vi "Swervepostprossesing(mine) (SubVI).vi"(7 "Total ticks in rotation":dbl, 9 "Speed in":dbl, 10 "Angle in":dbl, 11 "refnum name":string="Steering FR") -> (0 "Boolean":bool=TRUE, 1 "Speed out":dbl, 2 "position":dbl, 3 "refnum name":string="Steering FR")   [LabVIEW 2020]
uses:
  <vilib>/Rock Robotics/WPI/ThirdParty/Phoenix-LabVIEW/Motor Controller/Get/CTRE_Phoenix_MotorController_GetSelectedSensorData.vi
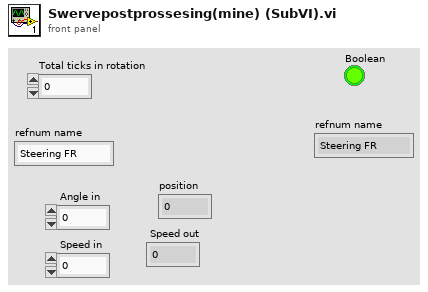
[diagram p1: front panel]
types:
  T1 = typedef "WPI_MotorControlDeviceRef.ctl" = cluster{"DeviceStatus":errorcluster, "Type":T2, "PWM":cluster{"PWM Channel":T3, "DeadBand":T4}, "CAN":cluster{"Device Number":u8, "SetOutput VI Ref":variant, "GetOutput VI Ref":variant, "Enable VI Ref":variant, "Disable VI Ref":variant, "Data":variant}, "Invert":bool, "DIO PWM":cluster{"PWM \"Enable\" Channel":T3, "DIOChannel":T5, "PWM Rate":dbl}}
  T2 = typedef "WPI_MotorControlType.ctl" = enum16{"PWM", "CAN", "DIO PWM"}
  T3 = typedef "FPGA_DIOPWMChannel.ctl" = enum8{"PWM 0", "PWM 1", "PWM 2", "PWM 3", "PWM 4", "PWM 5", "PWM 6", "PWM 7", "PWM 8", "PWM 9", "PWM MXP 0", "PWM MXP 1", "PWM MXP 2", "PWM MXP 3", "PWM MXP 4", "PWM MXP 5", "PWM MXP 6", "PWM MXP 7", "PWM MXP 8", "PWM MXP 9", "Invalid"}
  T4 = typedef "WPI_PWMDeadband.ctl" = cluster{"Name":string, "maxPositivePwm":i32, "minPositivePwm":i32, "centerPwm":i32, "maxNegativePwm":i32, "minNegativePwm":i32, "angularRange":u16}
  T5 = typedef "FPGA_DIOChannel.ctl" = enum8{"DIO 0", "DIO 1", "DIO 2", "DIO 3", "DIO 4", "DIO 5", "DIO 6", "DIO 7", "DIO 8", "DIO 9", "DIO MXP 0", "DIO MXP 1", "DIO MXP 2", "DIO MXP 3", "DIO MXP 4", "DIO MXP 5", "DIO MXP 6", "DIO MXP 7", "DIO MXP 8", "DIO MXP 9", "DIO MXP 10", "DIO MXP 11", "DIO MXP 12", "DIO MXP 13", "DIO MXP 14", "DIO MXP 15", "SPI Port CS1", "SPI Port CS2", "SPI Port CS3", "SPI Port MISO", "SPI Port MOSI", "Invalid"}
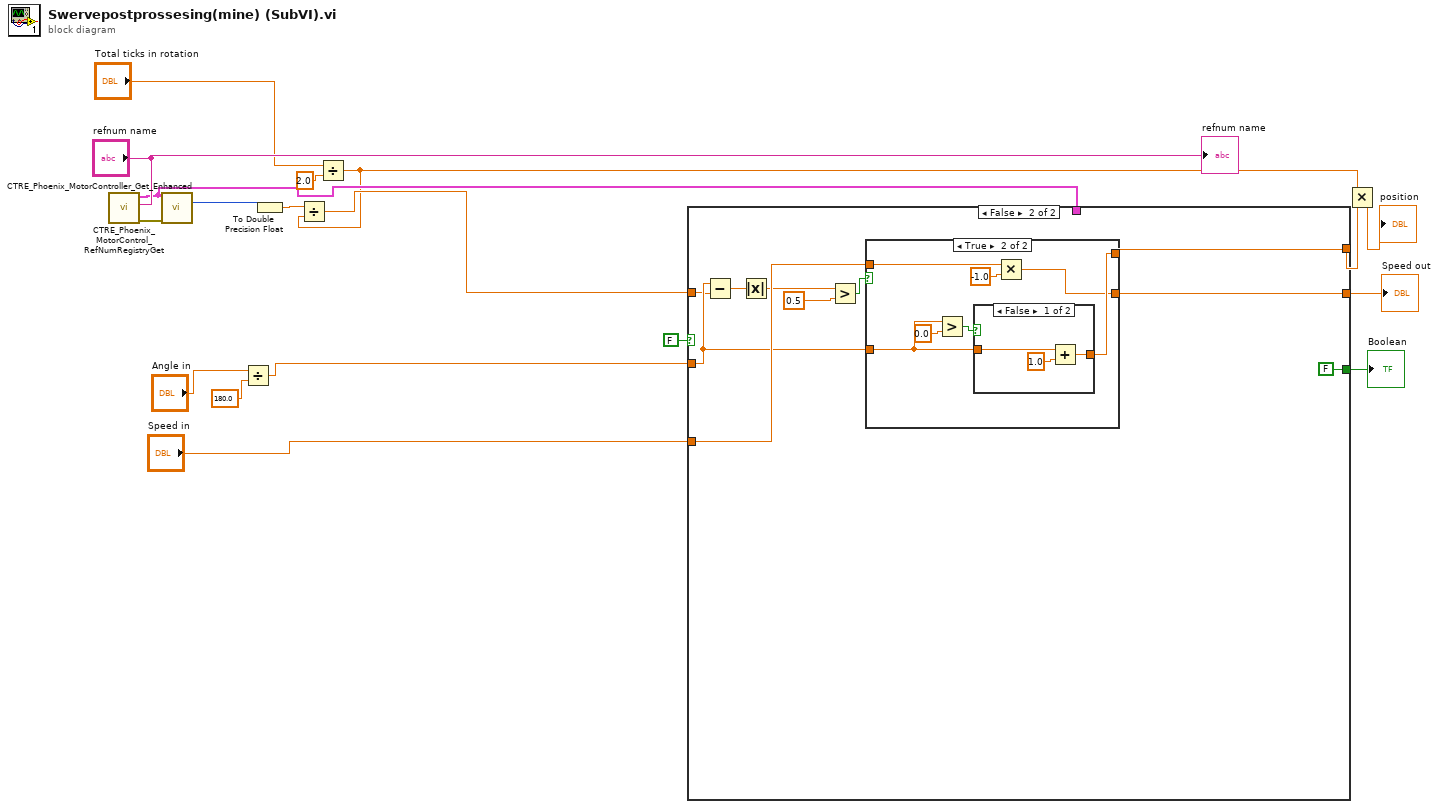
[diagram p0: block diagram]
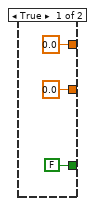
[diagram p2: hidden frame]
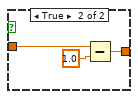
[diagram p4: hidden frame]
diagram:
  n1 = call <vilib>:"CTRE_Phoenix_MotorControl_RefNumRegistryGet.vi"("refnum name"="refnum name") -> ("error out"=w11:errorcluster, "PhoenixMotorControlDevRef"=w4:T1)  [unwired: 9 in]
  n2 = call-poly <vilib>:"CTRE_Phoenix_MotorController_Get_Enhanced.vi"("PhoenixMotorControlDevRef"=w4, "error in"=w11) -> ("Position (Raw Sensor Units)"=w14:i32)  [unwired: 10 in, 3 out]
  n3 = Divide(x="Angle in", y=180.0) -> (x/y=w8:dbl)
  n4 = To Double Precision Float(number=w14) -> (double precision float=w15:dbl)
  n5 = Divide(x="Total ticks in rotation", y=2.0) -> (x/y=w1:dbl)
  n6 = Divide(x=w15, y=w1) -> (x/y=w5:dbl)
  n7 = case shown="False" FALSE {
    tunnel: [0.0 ("Speed in") w31] -> w17
    tunnel: "Speed in" -> [_ w30]
    tunnel: w8 -> [_ w29]
    tunnel: w5 -> [_ w24]
    tunnel: [0.0 w23] -> w7
    tunnel: w4 -> [_ _]
    tunnel: [FALSE FALSE] -> w3
    frame True {
    }
    frame False {
      n8 = Subtract(x=w29, y=w24) -> (x-y=w25:dbl)
      n9 = Absolute Value(x=w25) -> (abs(x)=w27:dbl)
      n10 = Greater?(x=w27, y=0.5) -> (0:w28:bool)
      n11 = case shown="True" w28 {
        tunnel: w29 -> [w33 w38]
        tunnel: [w33 w37] -> w23
        tunnel: w30 -> [w32 w36]
        tunnel: [w32 w34] -> w31
        frame False {
        }
        frame True {
          n12 = Greater?(x=w38, y=0.0) -> (0:w39:bool)
          n13 = case shown="False" w39 {
            tunnel: w38 -> [w43 w46]
            tunnel: [w41 w44] -> w37
            frame False {
              n14 = Add(x=w43, y=1.0) -> (x+y=w41:dbl)
            }
            frame True {
              n15 = Subtract(x=w46, y=1.0) -> (x-y=w44:dbl)
            }
          }
          n16 = Multiply(x=w36, y=-1.0) -> (x*y=w34:dbl)
        }
      }
    }
  }
  "Speed out" <- w17
  "Boolean" <- w3
  n17 = Multiply(x=w1, y=w7) -> (x*y=→"position":dbl)
  "refnum name" <- "refnum name"
